vi "sub.vi"(11 "Numeric 3":i32) -> (2 "Numeric 2":i32)   [LabVIEW 2017]
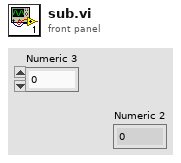
[diagram p1: front panel]
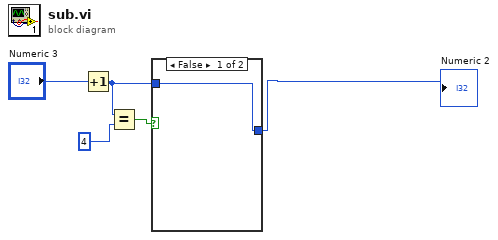
[diagram p0: block diagram]
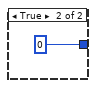
[diagram p2: hidden frame]
diagram:
  n1 = Increment(x="Numeric 3") -> (x+1=w5:i32)
  n2 = Equal?(x=w5, y=4) -> (x = y?=w3:bool)
  n3 = case shown="False" w3 {
    tunnel: [w6 0] -> w4
    tunnel: w5 -> [w6 _]
    frame False {
    }
    frame True {
    }
  }
  "Numeric 2" <- w4
